vi "MotionMacro@Go(Combine)__Parameter.vi"(1 "ParamterIn":string) -> (0 "ParamterOut":string)   [LabVIEW 2020]
panel:
  in  "Position":string(combo)
  in  "Speed":string(combo)
  in  "Axis":string(combo)
  in  "MotorName":string(combo)
  in  "Confirm":bool
  # "Motor@Go $Motor,$Axis,$Speed,$X(,$Y,$Z,$U...)"
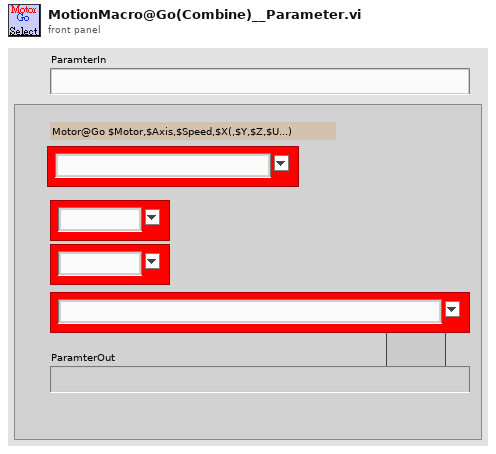
[diagram p1: front panel]
types:
  T1 = enum16{"Get", "Init", "Set", "Delete", "GetElement", "Inc", "Dec", "ReName", "Copy"}
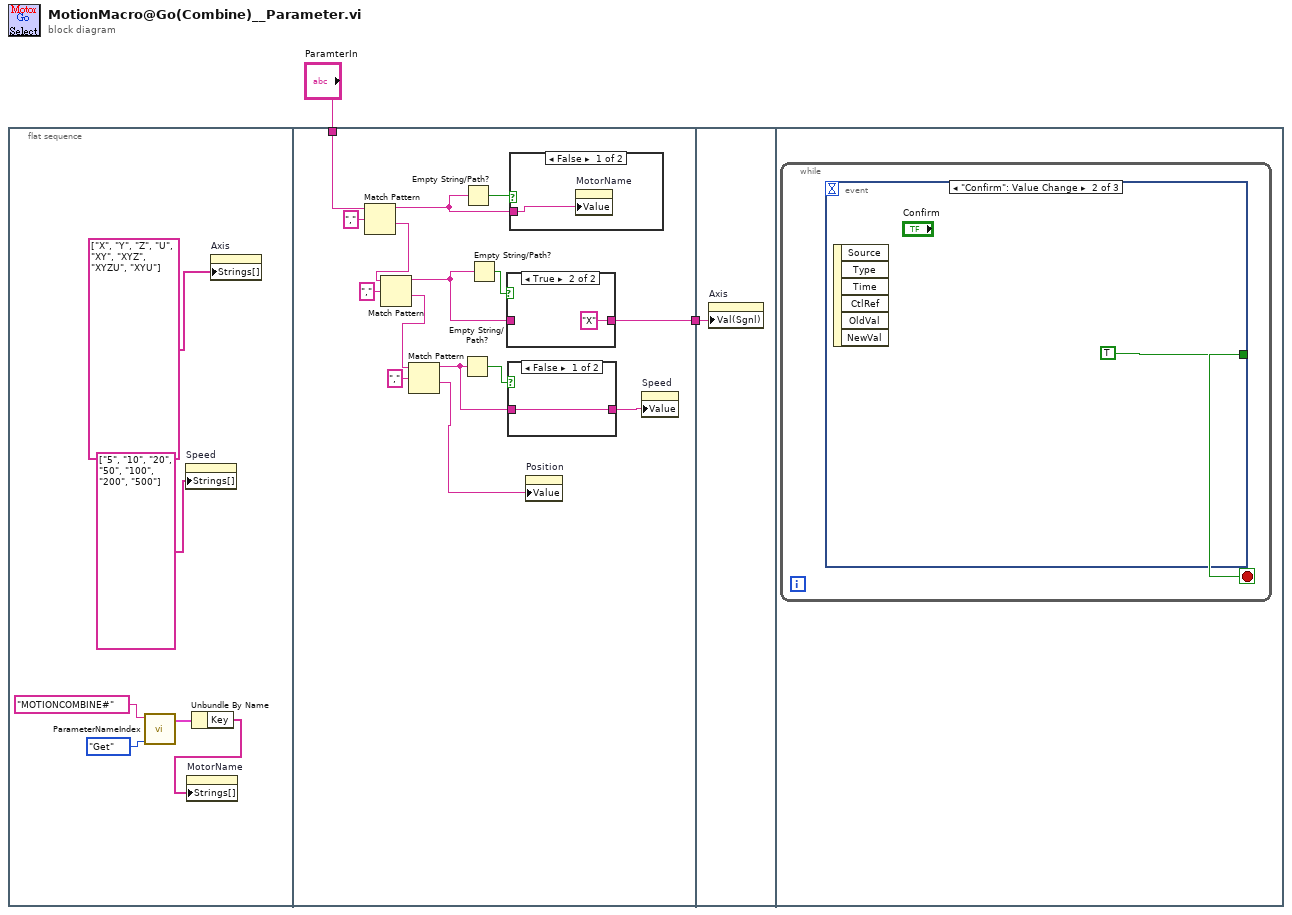
[diagram p0: block diagram]
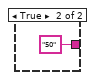
[diagram p2: hidden frame]
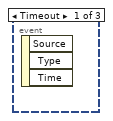
[diagram p5: hidden frame]
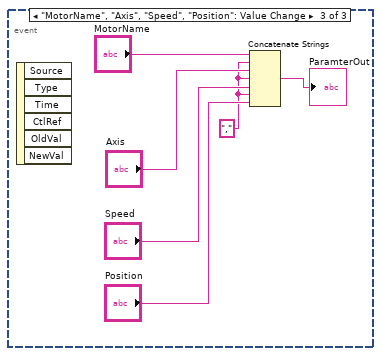
[diagram p6: hidden frame]
diagram:
  n1 = flat-sequence {
    tunnel: "ParamterIn" -> [w20]
    tunnel: [w21] -> w1
    tunnel: w1 -> [w29]
    frame #0 {
      n2 = call "ParameterNameIndex.vi"("OP"=T1."Get", "VariableSection"="MOTIONCOMBINE#" ("string")) -> ("SectionKeyValue"=w5:cluster{"Key":string[], "Value":string[]})  [unwired: 3 in, 6 out]
      n3 = property on="Speed" class="CmbBox"("Strings[]"=string[] ["5", "10", "20", "50", "100", "200", "500"] ("Strings []")) -> ()  [unwired: 2 in, 2 out]
      n4 = Unbundle By Name(w5) -> ("Key"=w4:string[])
      n5 = property on="MotorName" class="CmbBox"("Strings[]"=w4) -> ()  [unwired: 2 in, 2 out]
      n6 = property on="Axis" class="CmbBox"("Strings[]"=string[] ["X", "Y", "Z", "U", "XY", "XYZ", "XYZU", "XYU"] ("Strings []")) -> ()  [unwired: 2 in, 2 out]
    }
    frame #1 {
      n7 = Match Pattern(string=w20, regular expression="," ("search string")) -> (before substring=w18:string, after substring=w16:string)  [unwired: 1 in, 2 out]
      n8 = Match Pattern(string=w16, regular expression="," ("search string")) -> (before substring=w15:string, after substring=w13:string)  [unwired: 1 in, 2 out]
      n9 = Match Pattern(string=w13, regular expression="," ("search string")) -> (before substring=w9:string, after substring=w10:string)  [unwired: 1 in, 2 out]
      n10 = Empty String/Path?(string/path=w9) -> (empty?=w12:bool)
      n11 = Empty String/Path?(string/path=w18) -> (empty?=w23:bool)
      n12 = Empty String/Path?(string/path=w15) -> (empty?=w22:bool)
      n13 = case shown="True" w22 {
        tunnel: [w26 "X" ("ParamterIn")] -> w21
        tunnel: w15 -> [w26 _]
        frame False {
        }
        frame True {
        }
      }
      n14 = case shown="False" w12 {
        tunnel: [w24 "50" ("ParamterIn")] -> w11
        tunnel: w9 -> [w24 _]
        frame False {
        }
        frame True {
        }
      }
      n15 = case shown="False" w23 {
        tunnel: w18 -> [w28 _]
        frame False {
          n16 = property on="MotorName" class="CmbBox"("Value"=w28) -> ()  [unwired: 2 in, 2 out]
        }
        frame True {
        }
      }
      n17 = property on="Position" class="CmbBox"("Value"=w10) -> ()  [unwired: 2 in, 2 out]
      n18 = property on="Speed" class="CmbBox"("Value"=w11) -> ()  [unwired: 2 in, 2 out]
    }
    frame #2 {
      n19 = property on="Axis" class="CmbBox"("Val(Sgnl)"=w29) -> ()  [unwired: 2 in, 2 out]
    }
    frame #3 {
      n20 = while {
        stop <- w30 stop-if-true
        n21 = event shown="[1] \"Confirm\": Value Change" {
          selector: _ -> [_ _ _]
          dyn-events: _ -> [_ _ _]
          timeout: _ -> [_ _ _]
          tunnel: [_ TRUE _] -> w30
          event Timeout {
            n22 = event-data() -> ()  [unwired: 1 in, 3 out]
          }
          event "Confirm": Value Change {
            n23 = event-data() -> ()  [unwired: 1 in, 6 out]
          }
          event "MotorName", "Axis", "Speed", "Position": Value Change {
            w32 = "," ("string")
            n24 = event-data() -> ()  [unwired: 1 in, 6 out]
            n25 = Concatenate Strings("MotorName", w32, "Axis", w32, "Speed", w32, "Position") -> (→"ParamterOut":string)
          }
        }
      }
    }
  }
